vi "Main.vi"(8 "error in":errorcluster) -> (0 "error out":errorcluster)   [LabVIEW 2020]
uses:
  CLA ATM/Controller/Controls/Application Events.ctl
  CLA ATM/Controller/Controller.lvlib
  CLA ATM/Controller/Controls/Application Event Object.ctl
  CLA ATM/Error/Controls/Error Message Object.ctl
  CLA ATM/Error/Error Handler.lvlib
  CLA ATM/Controller/Controls/Application Modules.ctl
  CLA ATM/Display Console/Display Console.lvlib
  CLA ATM/User Console/User Console.lvlib
  CLA ATM/Sensor Interface/Sensor Interface.lvlib
  CLA ATM/Error/Controls/Error Commands.ctl
panel:
  in  "Use Simulated Sensor Interface":bool=TRUE
  in  "Use Simulated User Console":bool=TRUE
  in  "Use Simulated Display Console":bool=TRUE
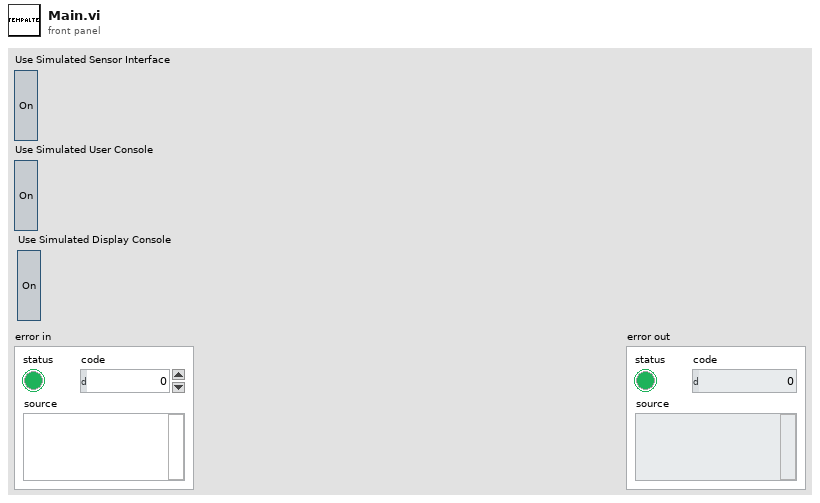
[diagram p1: front panel]
types:
  T1 = typedef "Error Handler.lvlib/Error Message Object.ctl" = cluster{"Source Module":T2, "Error":errorcluster, "Command":T3}
  T2 = typedef "Controller.lvlib/Application Modules.ctl" = enum16{"Controller", "Error Module", "User Console", "Display Console", "Sensor Interface"}
  T3 = typedef "Error Handler.lvlib/Error Commands.ctl" = enum16{"Stop", "Process Error", "Initialize"}
  T4 = typedef "Controller.lvlib/Application Event Object.ctl" = cluster{"Events":T5, "Source Module":T2, "Event Data":variant}
  T5 = typedef "Controller.lvlib/Application Events.ctl" = enum16{"Shutdown", "Initialize", "New Transaction", "Balance Inquiry", "Deposit", "Withdrawal", "Fast Cash 50$", "Terminate Session", "Login", "Verify Account"}
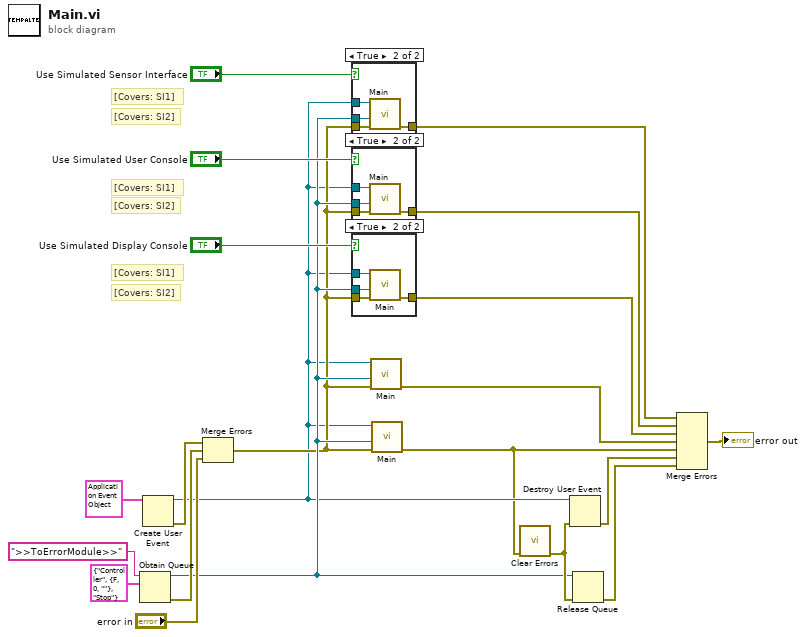
[diagram p0: block diagram]
diagram:
  # "[Covers: SI2]"
  # "[Covers: SI2]"
  # "[Covers: SI2]"
  # "[Covers: SI1]"
  # "[Covers: SI1]"
  # "[Covers: SI1]"
  n1 = Obtain Queue(name (unnamed)=">>ToErrorModule>>", element data type=T1 {"Source Module"=enum."Controller", "Error"={"status"=FALSE, "code"=0, "source"=""}, "Command"=enum."Stop"}) -> (queue out=w8:refnum<queue>, error out=w14:errorcluster)  [unwired: 3 in, 1 out]
  n2 = Create User Event(user event datatype=T4 {"Events"=enum."Shutdown", "Source Module"=enum."Controller", "Event Data"=variant} ("ApplicationEvents")) -> (user event=w6:refnum<user-event>, error out=w15:errorcluster)  [unwired: 1 in]
  n3 = Merge Errors(w15, w14, "error in") -> (w7:errorcluster)
  n4 = case shown="True" "Use Simulated Sensor Interface" {
    tunnel: w6 -> [_ w26]
    tunnel: w8 -> [_ w25]
    tunnel: w7 -> [w22 w24]
    tunnel: [w22 w23] -> w5
    frame False {
    }
    frame True {
      n5 = call "Main.vi"("error in"=w24, "Error Queue"=w25, "Application Events"=w26) -> ("error out"=w23:errorcluster)  [unwired: 8 in]
    }
  }
  n6 = case shown="True" "Use Simulated User Console" {
    tunnel: w6 -> [_ w31]
    tunnel: w8 -> [_ w30]
    tunnel: w7 -> [w27 w29]
    tunnel: [w27 w28] -> w4
    frame False {
    }
    frame True {
      n7 = call "Main.vi"("error in"=w29, "Error Queue"=w30, "Application Events"=w31) -> ("error out"=w28:errorcluster)  [unwired: 8 in]
    }
  }
  n8 = case shown="True" "Use Simulated Display Console" {
    tunnel: w6 -> [_ w36]
    tunnel: w8 -> [_ w35]
    tunnel: w7 -> [w32 w34]
    tunnel: [w32 w33] -> w11
    frame False {
    }
    frame True {
      n9 = call "Main.vi"("error in"=w34, "Error Queue"=w35, "Application Events"=w36) -> ("error out"=w33:errorcluster)  [unwired: 8 in]
    }
  }
  n10 = call "Main.vi"("error in"=w7, "Error Queue"=w8, "Application Events"=w6) -> ("error out"=w12:errorcluster)  [unwired: 8 in]
  n11 = call "Main.vi"("error in"=w7, "Error Queue"=w8, "Application Events"=w6) -> ("error out"=w1:errorcluster)  [unwired: 8 in]
  n12 = call <vilib>:"Clear Errors.vi"("error in (no error)"=w1) -> ("error out"=w17:errorcluster)  [unwired: 5 in, 1 out]
  n13 = Destroy User Event(user event=w6, error in=w17) -> (error out=w2:errorcluster)
  n14 = Release Queue(queue=w8, error in (no error)=w17) -> (error out=w3:errorcluster)  [unwired: 1 in, 2 out]
  n15 = Merge Errors(w5, w4, w11, w12, w1, w2, w3) -> (→"error out":errorcluster)
